vi "Outline Creater - Detects EQUALS.vi"() -> ()   [LabVIEW 2015]
uses:
  <vilib>/userdefined/High Color/IMAQdx.ctl
  <vilib>/vision/NI_Vision_Development_Module.lvlib
  <vilib>/vision/driver/NI_Vision_Acquisition_Software.lvlib
  <resource>/objmgr/imaqdx.rc
panel:
  out "Processed Image":T1(plugin-control)
  out "Image 2":T1(plugin-control)
  out "Image":T1(plugin-control)
  in  "Start Column":i32
  in  "Start Row":i32
  in  "stop":bool
  out "ARRAY SIZE":dbl[][](array[numeric])
  in  "Number of LED Array Variables":i32=160
  out "Video Modes":string
  in  "Video Mode":dbl min=0.0 max=5.0 step=1.0
  in  "Camera":T2
  out "Y Resoloution":i32
  out "X Resoloution":i32
  in  "error in (no error)":errorcluster
  out "error out":errorcluster
  in  "Threshold for LED Array":u8(slide)=100 step=5 scale=0.0..255.0
  out "LED Array/Outline":bool[][](array[boolean])
  out "Image Values":u8[][](array[numeric])
  in  "Stop 2":bool
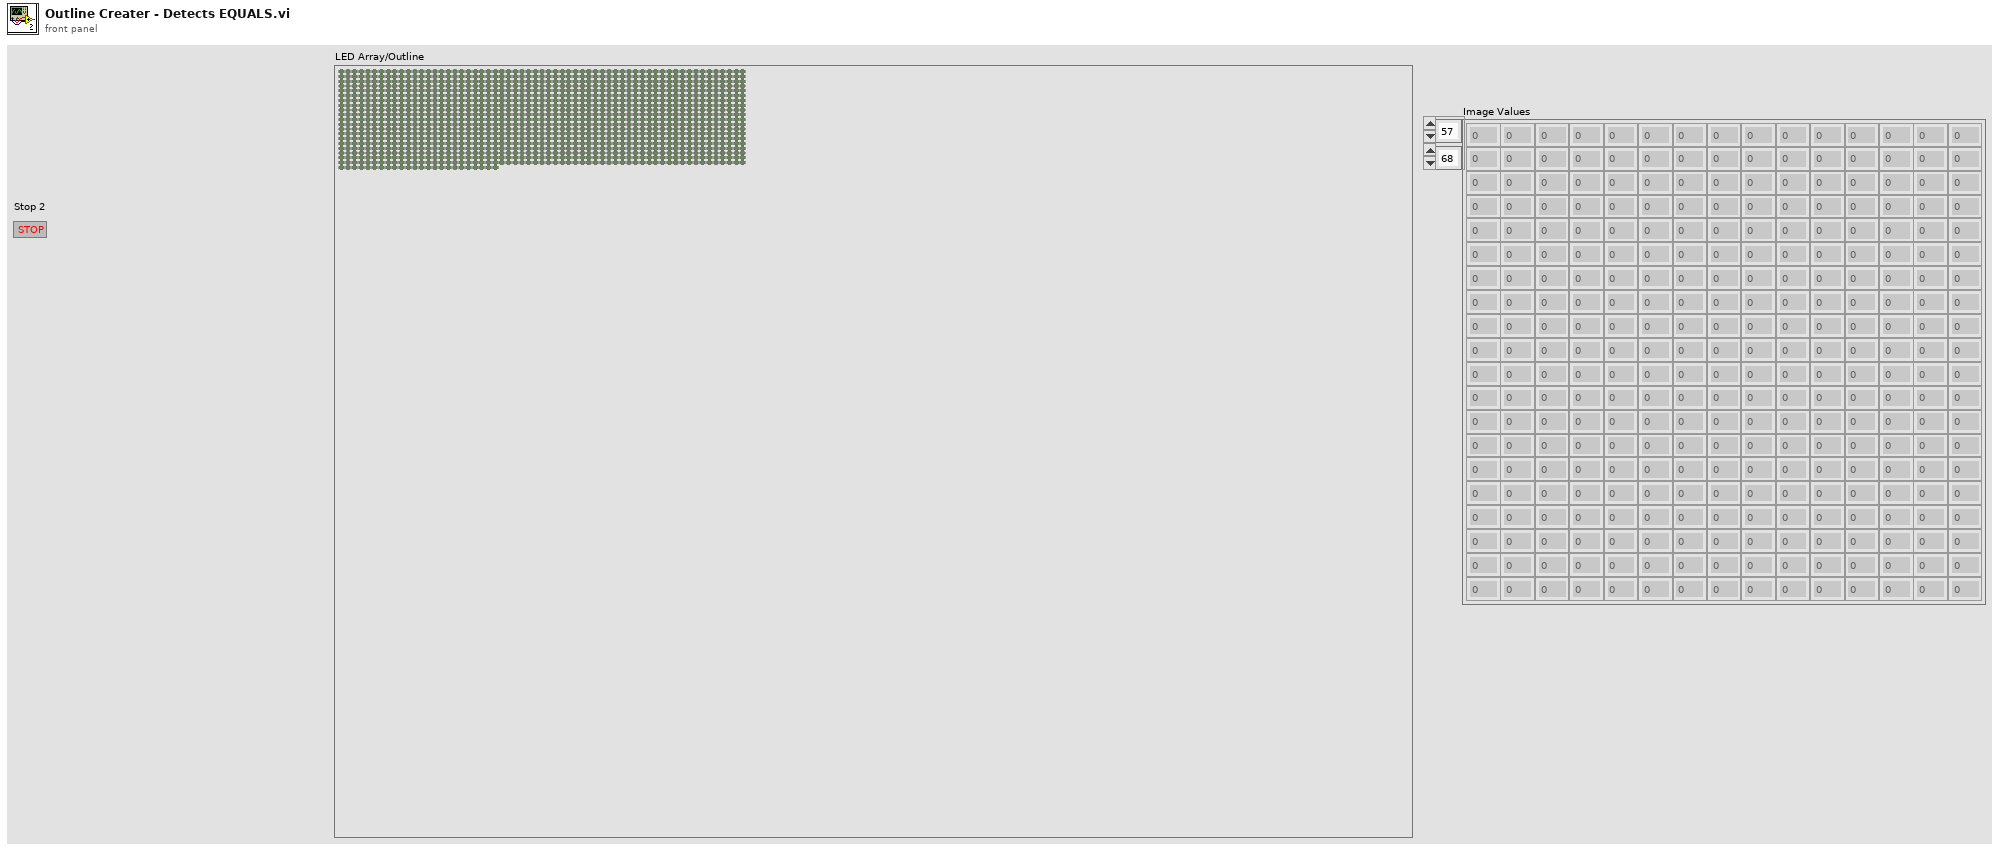
[diagram p1: front panel]
types:
  T1 = typedef "IMAQ Image.ctl" = refnum<image>
  T2 = typedef "IMAQdx.ctl" = refnum<k21>
  T3 = typedef "IMAQ Circle" = cluster{"Center X":i32, "Center Y":i32, "Inner Radius":i32, "Outer Radius":i32, "Start Angle":dbl, "End Angle":dbl}
  T4 = cluster{"Center":cluster{"X":sgl, "Y":sgl}, "Radius":dbl}
  T5 = typedef "ROI Descriptor" = cluster{"Global Rectangle":i32[], "Contours":cluster{"ID":enum32{"External", "Internal"}, "Type":u32, "Coordinates":i32[]}[]}
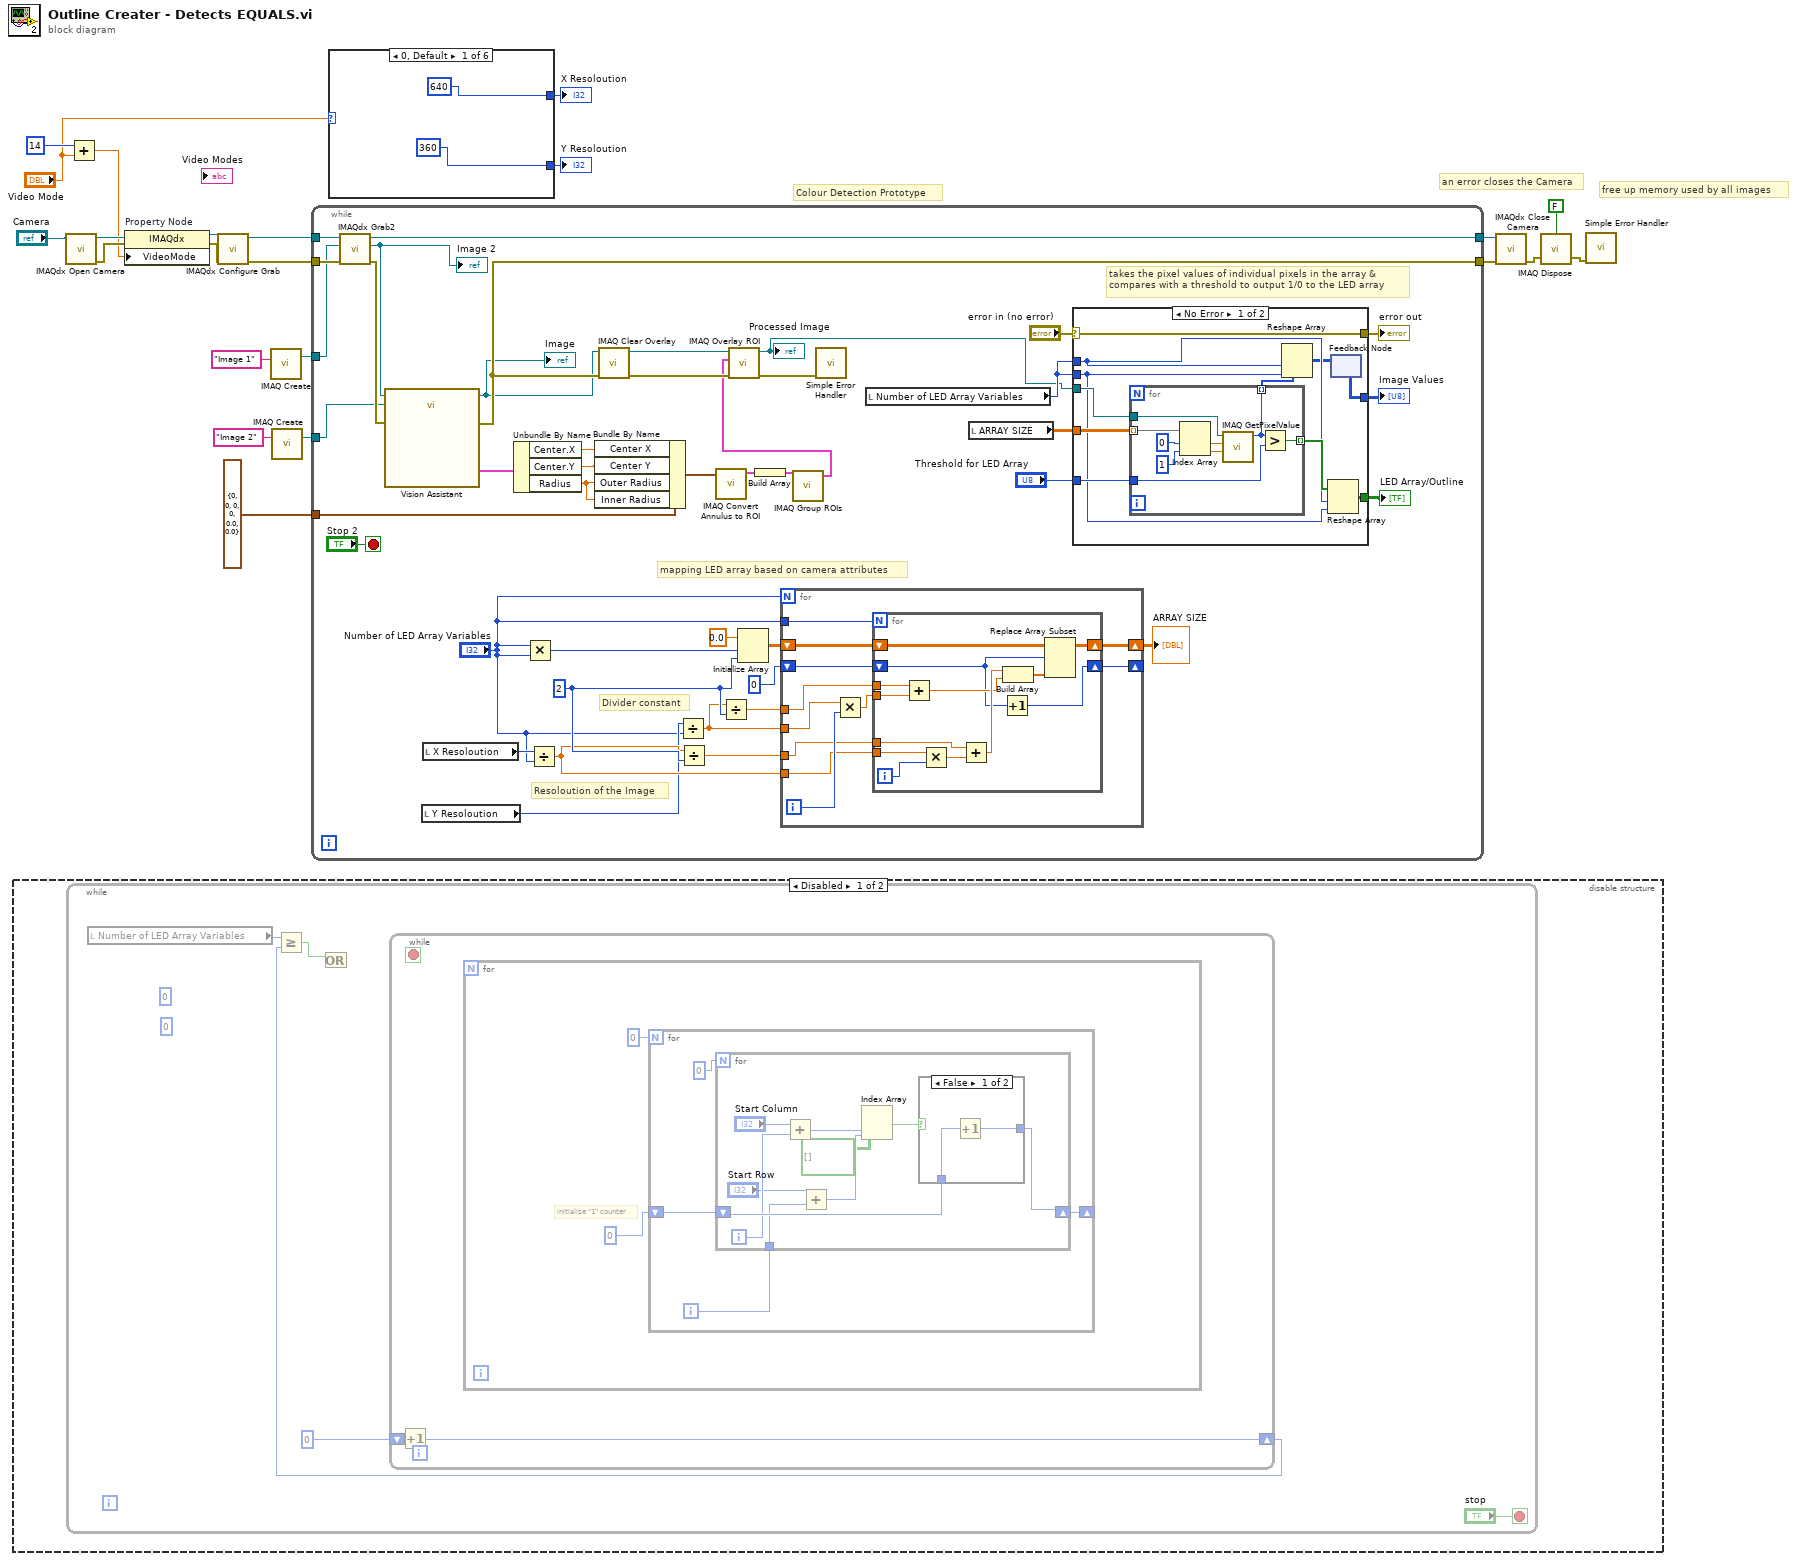
[diagram p0: block diagram]
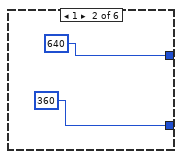
[diagram p4: hidden frame]
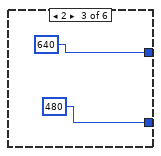
[diagram p5: hidden frame]
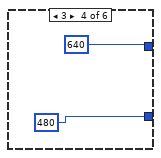
[diagram p6: hidden frame]
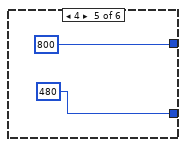
[diagram p7: hidden frame]
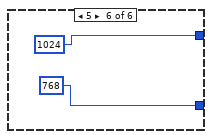
[diagram p8: hidden frame]
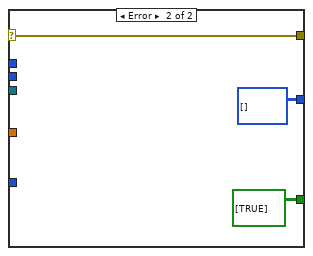
[diagram p9: hidden frame]
diagram:
  # "Colour Detection Prototype"
  # "an error closes the Camera"
  # "free up memory used by all images"
  n1 = disable-structure shown="Disabled" {
    frame Disabled {
      n2 = while {
        stop <- "stop" stop-if-true
        (unwired) 0
        (unwired) 0
        n3 = local read "Number of LED Array Variables"() -> (w25:i32)
        n4 = while {
          shift-right: [w28] -> w26
          shift-left: 0 ("Numeric") -> [w29]
          stop <- _ stop-if-true
          n5 = Increment(x=w29) -> (x+1=w28:i32)
          n6 = for {
            # "initialise \"1\" counter"
            n7 = for {
              N: 0 -> [_]
              shift-right: [w34] -> _
              shift-left: 0 -> [w35]
              i -> [w33]
              n8 = for {
                N: 0 -> [_]
                shift-right: [w44] -> w34
                shift-left: w35 -> [w45]
                tunnel: w33 -> [w37]
                i -> [w42]
                n9 = Add(x="Start Column", y=w42) -> (x+y=w40:i32)
                n10 = Add(x="Start Row", y=w37) -> (x+y=w38:i32)
                n11 = Index Array(array=bool[][] [], index (row)=w40, index (col)=w38) -> (element=w43:bool)
                n12 = case shown="False" w43 {
                  tunnel: w45 -> [w46 w48]
                  tunnel: [w47 w48] -> w44
                  frame False {
                    n13 = Increment(x=w46) -> (x+1=w47:i32)
                  }
                  frame True {
                  }
                }
              }
            }
          }
        }
        n14 = Greater Or Equal?(x=w25, y=w26) -> (x >= y?=w23:bool)
        n15 = Or(x=w23) -> ()  [unwired: 1 in, 1 out]
      }
    }
    frame Enabled {
    }
  }
  n16 = call <vilib>:"IMAQdx Open Camera.vi"("Session In"="Camera") -> ("error out"=w12:errorcluster, "Session Out"=w13:T2)  [unwired: 9 in]
  n17 = Add(x=14, y="Video Mode") -> (x+y=w7:dbl)
  n18 = property on="Property Node" class="IMAQdx"(reference=w13, error in=w12, "VideoMode"=w7) -> (reference out=w11:T2, error out=w10:errorcluster)
  n19 = call <vilib>:"IMAQdx Configure Grab.vi"("error in"=w10, "Session In"=w11) -> ("error out"=w1:errorcluster, "Session Out"=w2:T2)  [unwired: 8 in]
  n20 = call "IMAQ Create"("Image Name"="Image 1") -> ("New Image"=w16:T1)  [unwired: 4 in, 1 out]
  n21 = call "IMAQ Create"("Image Name"="Image 2") -> ("New Image"=w19:T1)  [unwired: 4 in, 1 out]
  n22 = while {
    tunnel: [w53] -> w15
    tunnel: w19 -> [w49]
    tunnel: w1 -> [w77]
    tunnel: w2 -> [w76]
    tunnel: w16 -> [w75]
    tunnel: [w74] -> w14
    tunnel: T3 {"Center X"=0, "Center Y"=0, "Inner Radius"=0, "Outer Radius"=0, "Start Angle"=0.0, "End Angle"=0.0} ("Annulus") -> [w58]
    stop <- "Stop 2" stop-if-true
    w85 = 2
    # "takes the pixel values of individual pixels in the array & \ncompares with a threshold to output 1/0 to the LED array"
    # "mapping LED array based on camera attributes"
    # "Divider constant"
    # "Resoloution of the Image"
    n23 = call <vilib>:"IMAQdx Grab2.vi"("error in"=w77, "Image In"=w75, "Session In"=w76) -> ("error out"=w66:errorcluster, "Image Out"=w65:T1, "Session Out"=w74:T2)  [unwired: 5 in, 1 out]
    "Image 2" <- w65
    n24 = call "Vision Assistant"("Image In"=w65, "Image Dst"=w49, "error in"=w66) -> ("Image Out"=w51:T1, "Best Circle (Fit Circle Ball 1)"=w60:T4, "error out"=w53:errorcluster)  [unwired: 1 in, 21 out]
    "Image" <- w51
    n25 = local read "Y Resoloution"() -> (w71:i32)
    n26 = local read "X Resoloution"() -> (w72:i32)
    n27 = Unbundle By Name(w60) -> ("Center.X"=w52:sgl, "Center.Y"=w61:sgl, "Radius"=w64:dbl)
    n28 = Multiply(x="Number of LED Array Variables", y="Number of LED Array Variables") -> (x*y=w86:i32)
    n29 = Divide(x=w72, y="Number of LED Array Variables") -> (x/y=w84:dbl)
    n30 = Bundle By Name(cluster=w58, "Center X"=w52, "Center Y"=w61, "Outer Radius"=w64, "Inner Radius"=w64) -> (w59:T3)
    n31 = call "IMAQ Clear Overlay"("error in (no error)"=w53, "Image"=w51) -> ("error out"=w56:errorcluster, "Image Out"=w55:T1)  [unwired: 1 in, 7 out]
    n32 = Divide(x=w71, y="Number of LED Array Variables") -> (x/y=w83:dbl)
    n33 = Divide(x=w84, y=w85) -> (x/y=w82:dbl)
    n34 = call "IMAQ Convert Annulus to ROI"("Annulus"=w59) -> ("ROI Descriptor"=w62:T5)  [unwired: 1 in, 8 out]
    n35 = Divide(x=w83, y=w85) -> (x/y=w81:dbl)
    n36 = Initialize Array(0.0 ("element"), w86, w85) -> (w87:dbl[][])
    n37 = Build Array(w62) -> (w63:T5[])
    n38 = for {
      N: "Number of LED Array Variables" -> [_]
      shift-right: [w97] -> _
      shift-left: 0 -> [w100]
      shift-right: [w98] -> w68
      shift-left: w87 -> [w99]
      tunnel: "Number of LED Array Variables" -> [w96]
      tunnel: w84 -> [w95]
      tunnel: w83 -> [w94]
      tunnel: w82 -> [w93]
      tunnel: w81 -> [w92]
      i -> [w102]
      n39 = Multiply(x=w94, y=w102) -> (x*y=w101:dbl)
      n40 = for {
        N: w96 -> [_]
        tunnel: w101 -> [w111]
        shift-right: [w106] -> w97
        shift-left: w100 -> [w107]
        shift-right: [w109] -> w98
        shift-left: w99 -> [w110]
        tunnel: w95 -> [w105]
        tunnel: w93 -> [w104]
        tunnel: w92 -> [w103]
        i -> [w115]
        n41 = Add(x=w103, y=w111) -> (x+y=w113:dbl)
        n42 = Multiply(x=w105, y=w115) -> (x*y=w112:dbl)
        n43 = Add(x=w104, y=w112) -> (x+y=w114:dbl)
        n44 = Increment(x=w107) -> (x+1=w106:i32)
        n45 = Build Array(w114, w113) -> (w108:dbl[])
        n46 = Replace Array Subset(array=w110, new element=w108, index (row)=w107) -> (w109:dbl[][])  [unwired: 1 in]
      }
    }
    "ARRAY SIZE" <- w68
    n47 = call "IMAQ Group ROIs"("ROI Descriptors"=w63) -> ("ROI Descriptor out"=w54:T5)  [unwired: 1 in, 3 out]
    n48 = call "IMAQ Overlay ROI"("error in (no error)"=w56, "ROI Descriptor"=w54, "Image"=w55) -> ("error out"=w57:errorcluster, "Image Out"=w50:T1)  [unwired: 3 in, 4 out]
    "Processed Image" <- w50
    n49 = call <vilib>:"Simple Error Handler.vi"("error in (no error)"=w57) -> ()  [unwired: 1 in, 8 out]
    n50 = local read "Number of LED Array Variables"() -> (w69:i32)
    n51 = local read "ARRAY SIZE"() -> (w67:dbl[][])
    n52 = case shown="No Error" "error in (no error)" {
      selector: "error in (no error)" -> [w126 w138]
      tunnel: [w126 w138] -> w79
      tunnel: w50 -> [w125 _]
      tunnel: "Threshold for LED Array" -> [w124 _]
      tunnel: [w122 bool[][] [[TRUE]]] -> w78
      tunnel: w67 -> [w123 _]
      tunnel: w69 -> [w120 _]
      tunnel: w69 -> [w119 _]
      tunnel: [w117 u8[][] []] -> w80
      frame No Error {
        n53 = for {
          tunnel: w123 -> [w127] mode=indexing
          tunnel: w125 -> [w133]
          tunnel: [w130] -> w121 mode=indexing
          tunnel: w124 -> [w129]
          tunnel: [w128] -> w116 mode=indexing
          n54 = Index Array(array=w127, index #1=0 ("index"), index #2=1 ("index")) -> (element #1=w132:dbl, element #2=w131:dbl)
          n55 = call "IMAQ GetPixelValue"("Image"=w133, "X Coordinate"=w132, "Y Coordinate"=w131) -> ("Pixel Value (U8)"=w128:u8)  [unwired: 3 in, 4 out]
          n56 = Greater?(x=w128, y=w129) -> (0:w130:bool)
        }
        n57 = Reshape Array(w116, w120, w119) -> (w118:u8[][])
        n58 = Reshape Array(w121, w120, w119) -> (w122:bool[][])
        n59 = feedback-in #1(w118) -> ()
        n60 = feedback #1() -> (w117:u8[][])  [unwired: 1 in]
      }
      frame Error {
      }
    }
    "error out" <- w79
    "LED Array/Outline" <- w78
    "Image Values" <- w80
  }
  n61 = case shown="0, Default" "Video Mode" {
    tunnel: [640 640 640 640 800 1024] -> w4
    tunnel: [360 360 480 480 480 768] -> w5
    frame 0, Default {
    }
    frame 1 {
    }
    frame 2 {
    }
    frame 3 {
    }
    frame 4 {
    }
    frame 5 {
    }
  }
  "X Resoloution" <- w4
  "Y Resoloution" <- w5
  n62 = call <vilib>:"IMAQdx Close Camera.vi"("error in"=w15, "Session In"=w14) -> ("error out"=w20:errorcluster)  [unwired: 9 in]
  n63 = call "IMAQ Dispose"("All Images? (No)"=FALSE, "error in (no error)"=w20) -> ("error out"=w21:errorcluster)  [unwired: 4 in]
  n64 = call <vilib>:"Simple Error Handler.vi"("error in (no error)"=w21) -> ()  [unwired: 4 in, 5 out]
